vi "Configure Lights.vi"(8 "error in (no error)":errorcluster, 10 "Light Property":T1, 11 "Root Object In":refnum<vi>) -> (0 "error out":errorcluster, 3 "Root Object Out":refnum<vi>)   [LabVIEW 2020, in "3D Plot.lvclass"]
uses:
  3D Plot.lvclass
  Light Property.ctl
  Light Specific.ctl
  NI_3D Picture Control.lvlib
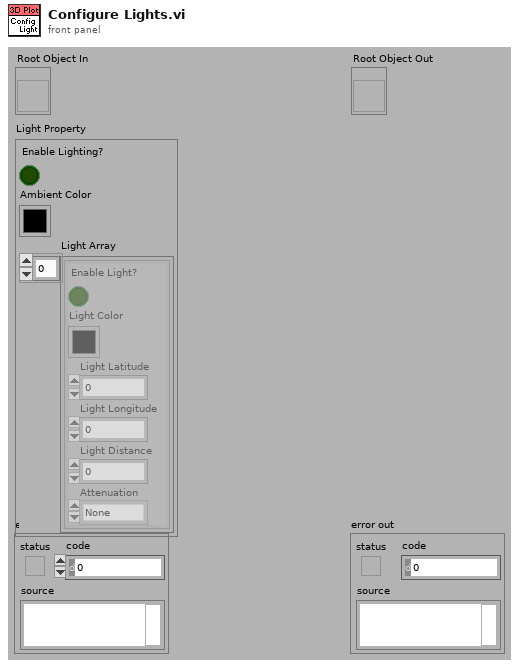
[diagram p1: front panel]
types:
  T1 = typedef "3D Plot.lvclass/Light Property.ctl" = cluster{"Enable Lighting?":bool, "Ambient Color":u32, "Light Array":T2[]}
  T2 = typedef "3D Plot.lvclass/Light Specific.ctl" = cluster{"Enable Light?":bool, "Light Color":u32, "Light Latitude":sgl, "Light Longitude":sgl, "Light Distance":sgl, "Attenuation":enum16{"None", "Linear", "Quadratic"}}
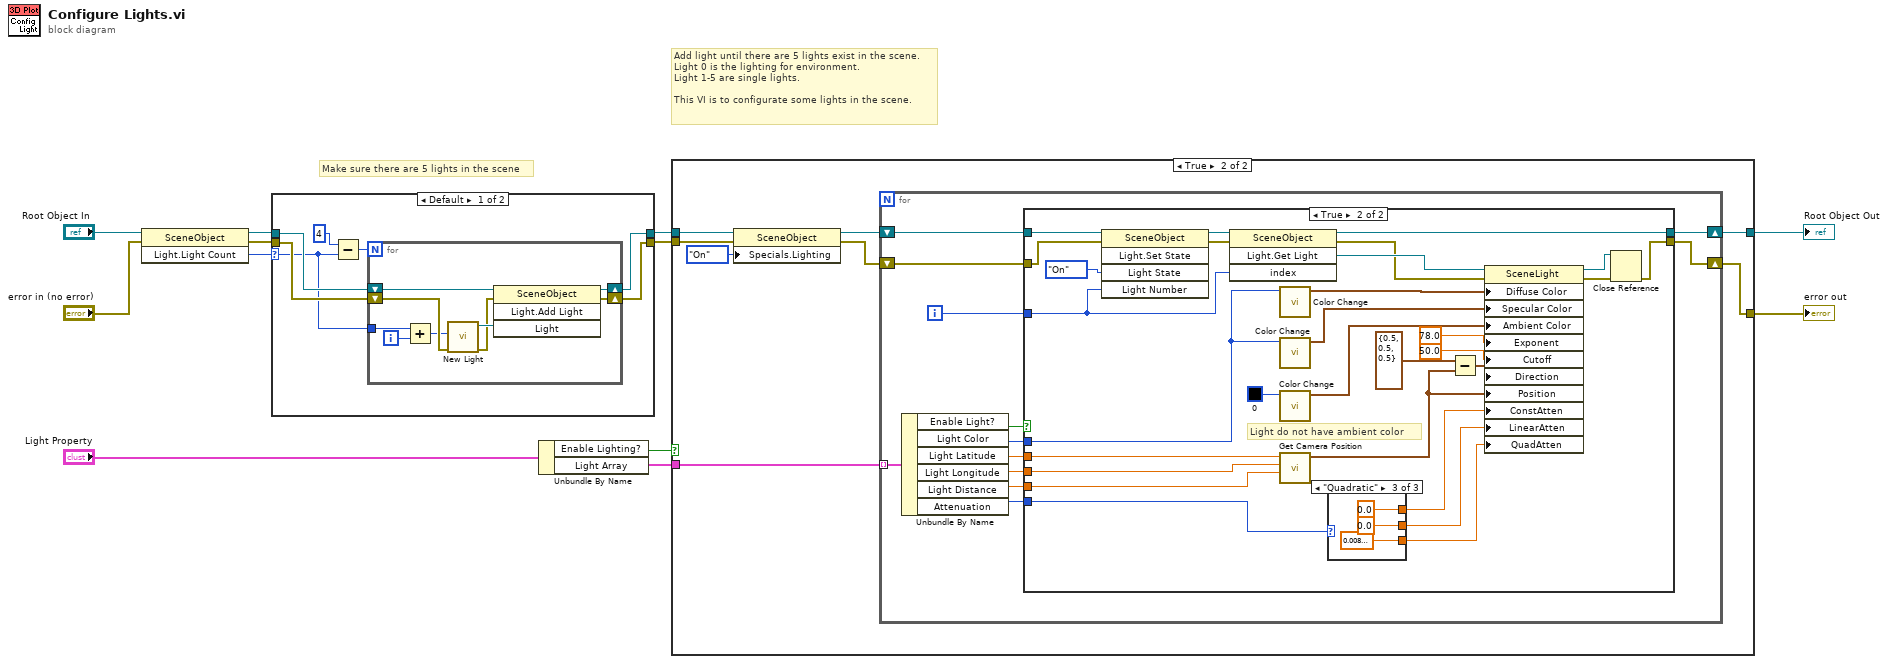
[diagram p0: block diagram]
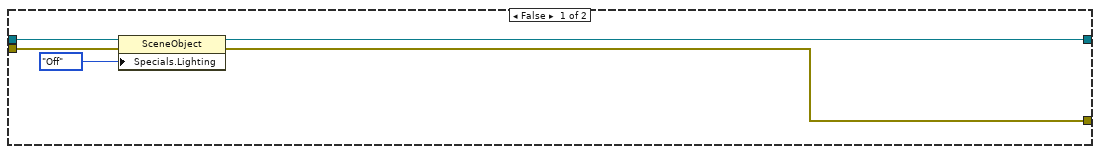
[diagram p3: hidden frame]
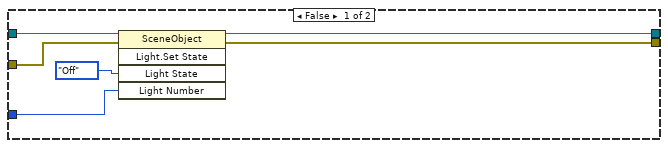
[diagram p4: hidden frame]
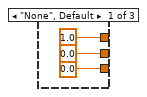
[diagram p5: hidden frame]
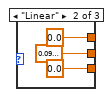
[diagram p6: hidden frame]
diagram:
  # "Make sure there are 5 lights in the scene"
  # "Add light until there are 5 lights exist in the scene.\nLight 0 is the lighting for environment.\nLight 1-5 are single lights.\n\nThis VI is to configurate some lights in the scene."
  n1 = invoke class="SceneObject" method="Light.Light Count"(reference="Root Object In", error in="error in (no error)") -> (reference out=w4:refnum<vi>, error out=w5:errorcluster, "Light Count"=w3:i32)  [unwired: 1 in]
  n2 = case shown="Default" w3 {
    selector: w3 -> [w13 _]
    tunnel: w5 -> [w19 w29]
    tunnel: w4 -> [w18 w30]
    tunnel: [w15 w30] -> w2
    tunnel: [w14 w29] -> w1
    frame Default {
      n3 = Subtract(x=4, y=w13) -> (x-y=w16:i32)
      n4 = for {
        N: w16 -> [_]
        shift-right: [w28] -> w15
        shift-left: w18 -> [w25]
        shift-right: [w27] -> w14
        shift-left: w19 -> [w24]
        tunnel: w13 -> [w21]
        i -> [w22]
        n5 = Add(x=w21, y=w22) -> (x+y=w20:i32)
        n6 = call "New Light.vi"("error in (no error)"=w24, "Light Number"=w20) -> ("error out"=w23:errorcluster, "New Light Refnum"=w26:refnum<vi>)  [unwired: 1 in, 7 out]
        n7 = invoke class="SceneObject" method="Light.Add Light"(reference=w25, error in=w23, "Light"=w26) -> (reference out=w28:refnum<vi>, error out=w27:errorcluster)  [unwired: 1 in, 2 out]
      }
    }
    frame 5 {
    }
  }
  n8 = Unbundle By Name("Light Property") -> ("Enable Lighting?"=w7:bool, "Light Array"=w6:T2[])
  n9 = case shown="True" w7 {
    tunnel: [w31 w43] -> w10
    tunnel: [w33 w41] -> w12
    tunnel: w2 -> [w34 w40]
    tunnel: w1 -> [w32 w38]
    tunnel: w6 -> [_ w42]
    frame False {
      n10 = property class="SceneObject"(reference=w34, error in=w32, "Specials.Lighting"=enum16{"Inherit Value", "Off", "On"}."Off" ("Specials:Lighting")) -> (reference out=w33:refnum<vi>, error out=w31:errorcluster)
    }
    frame True {
      n11 = property class="SceneObject"(reference=w40, error in=w38, "Specials.Lighting"=enum16{"Inherit Value", "Off", "On"}."On" ("Specials:Lighting")) -> (reference out=w37:refnum<vi>, error out=w36:errorcluster)
      n12 = for {
        shift-right: [w55] -> w43
        shift-left: w36 -> [w53]
        tunnel: w42 -> [w52] mode=indexing
        shift-right: [w45] -> w41
        shift-left: w37 -> [w54]
        i -> [w44]
        n13 = Unbundle By Name(w52) -> ("Enable Light?"=w50:bool, "Light Color"=w51:u32, "Light Latitude"=w49:sgl, "Light Longitude"=w48:sgl, "Light Distance"=w47:sgl, "Attenuation"=w46:enum16{"None", "Linear", "Quadratic"})
        n14 = case shown="True" w50 {
          tunnel: [w58 w62] -> w55
          tunnel: [w59 w66] -> w45
          tunnel: w54 -> [w61 w73]
          tunnel: w53 -> [w60 w72]
          tunnel: w51 -> [_ w65]
          tunnel: w44 -> [w57 w70]
          tunnel: w49 -> [_ w85]
          tunnel: w48 -> [_ w84]
          tunnel: w47 -> [_ w83]
          tunnel: w46 -> [_ w82]
          frame False {
            n15 = invoke class="SceneObject" method="Light.Set State"(reference=w61, error in=w60, "Light State"=enum16{"Inherit Value", "Off", "On"}."Off", "Light Number"=w57) -> (reference out=w59:refnum<vi>, error out=w58:errorcluster)  [unwired: 1 in, 3 out]
          }
          frame True {
            # "Light do not have ambient color"
            n16 = invoke class="SceneObject" method="Light.Set State"(reference=w73, error in=w72, "Light State"=enum16{"Inherit Value", "Off", "On"}."On", "Light Number"=w70) -> (reference out=w71:refnum<vi>, error out=w67:errorcluster)  [unwired: 1 in, 3 out]
            n17 = invoke class="SceneObject" method="Light.Get Light"(reference=w71, error in=w67, "index"=w70) -> (reference out=w66:refnum<vi>, error out=w68:errorcluster, "Get Light"=w69:refnum<vi>)  [unwired: 1 in, 1 out]
            n18 = call "Color Change.vi"("Color"=w65) -> ("RGBA"=w90:cluster{"R":sgl, "G":sgl, "B":sgl, "A":sgl})  [unwired: 1 in, 9 out]
            n19 = call "Color Change.vi"("Color"=w65) -> ("RGBA"=w88:cluster{"R":sgl, "G":sgl, "B":sgl, "A":sgl})  [unwired: 1 in, 9 out]
            n20 = call "Color Change.vi"("Color"=u32 0) -> ("RGBA"=w89:cluster{"R":sgl, "G":sgl, "B":sgl, "A":sgl})  [unwired: 1 in, 9 out]
            n21 = call "Get Camera Position.vi"("Distance"=w83, "Longitude"=w84, "Latitude"=w85) -> ("Camera Position"=w76:cluster{"X":sgl, "Y":sgl, "Z":sgl})  [unwired: 1 in, 7 out]
            n22 = case shown="\"Quadratic\"" w82 {
              tunnel: [sgl 0.0 ("Exponent") sgl 0.09 ("Exponent") sgl 0.0 ("Exponent")] -> w81
              tunnel: [sgl 0.0 ("Cutoff") sgl 0.0 ("Cutoff") sgl 0.008 ("Cutoff")] -> w80
              tunnel: [sgl 1.0 ("Attenuation:Constant Attenuation") sgl 0.0 ("Exponent") sgl 0.0 ("Exponent")] -> w79
              frame "None", Default {
              }
              frame "Linear" {
              }
              frame "Quadratic" {
              }
            }
            n23 = Subtract(x=cluster{"X":sgl, "Y":sgl, "Z":sgl} {"X"=0.5, "Y"=0.5, "Z"=0.5} ("Direction"), y=w76) -> (x-y=w75:cluster{"X":sgl, "Y":sgl, "Z":sgl})
            n24 = property class="SceneLight"(reference=w69, error in=w68, "Diffuse Color"=w90, "Specular Color"=w88, "Ambient Color"=w89, "Exponent"=sgl 78.0, "Cutoff"=sgl 50.0, "Direction"=w75, "Position"=w76, "ConstAtten"=w79, "LinearAtten"=w81, "QuadAtten"=w80) -> (reference out=w64:refnum<vi>, error out=w63:errorcluster)
            n25 = Close Reference(reference=w64, error in (no error)=w63) -> (error out=w62:errorcluster)
          }
        }
      }
    }
  }
  "error out" <- w10
  "Root Object Out" <- w12
